vi "rszvl_core_global.vi"() -> ()   [LabVIEW 2014] (continued)
"*WAI"=FALSE}, "Check Status Callback"=""}, {"Level"=2, "Descriptive Name"="Time Trigger", "Class Only"=TRUE, "Data Type"=0, "Access"=0, "Identifier"="", "Range Table"="", "Command"="", "Read Callback"="", "Write Callback"="", "Range Callback"="", "Check Callback"="", "Rngtable Callback"="", "Coerce Callback"="", "User Callback"="", "Supported Models"="", "Instrument Options"="", "Repeated Capabilities"="", "Restricted Repeated Capabilities"="", "Help"="Time Trigger configuration.\n\n(1) Time Interval:\nThis attribute sets the time intervall for the time trigger source.", "Flags"={"OPC Wait"=FALSE, "Dont check status"=FALSE, "*WAI"=FALSE}, "Check Status Callback"=""}, {"Level"=3, "Descriptive Name"="Time Interval", "Class Only"=FALSE, "Data Type"=1, "Access"=2, "Identifier"="RSZVL_ATTR_TRIGGER_TIME_INTERVAL", "Range Table"="rszvl_rngTriggerTimeInterval", "Command"="TRIG:TIME:RINT", "Read Callback"="", "Write Callback"="", "Range Callback"="", "Check Callback"="", "Rngtable Callback"="", "Coerce Callback"="", "User Callback"="", "Supported Models"="", "Instrument Options"="", "Repeated Capabilities"="", "Restricted Repeated Capabilities"="", "Help"="This attribute sets the time intervall for the time trigger source.\n\nAvailable Repeated Capabilities:\nNone\n\nRemote-control command(s):\nTRIGger<1|2>[:SEQuence]:TIME:RINTerval", "Flags"={"OPC Wait"=FALSE, "Dont check status"=FALSE, "*WAI"=FALSE}, "Check Status Callback"=""}, {"Level"=1, "Descriptive Name"="Amplitude", "Class Only"=TRUE, "Data Type"=0, "Access"=0, "Identifier"="", "Range Table"="", "Command"="", "Read Callback"="", "Write Callback"="", "Range Callback"="", "Check Callback"="", "Rngtable Callback"="", "Coerce Callback"="", "User Callback"="", "Supported Models"="", "Instrument Options"="", "Repeated Capabilities"="", "Restricted Repeated Capabilities"="", "Help"="(1) Amplitude Preamplifier State:\nThis attribute switches on the preamplifier for the instrument. The switchable gain is fixed to 20 dB.", "Flags"={"OPC Wait"=FALSE, "Dont check status"=FALSE, "*WAI"=FALSE}, "Check Status Callback"=""}, {"Level"=2, "Descriptive Name"="Amplitude Preamplifier State", "Class Only"=FALSE, "Data Type"=3, "Access"=2, "Identifier"="RSZVL_ATTR_AMPL_PREAMPLIFIER", "Range Table"="", "Command"="INP:GAIN:STAT", "Read Callback"="", "Write Callback"="", "Range Callback"="", "Check Callback"="", "Rngtable Callback"="", "Coerce Callback"="", "User Callback"="", "Supported Models"="", "Instrument Options"="", "Repeated Capabilities"="", "Restricted Repeated Capabilities"="", "Help"="This attribute switches on the preamplifier for the instrument. The switchable gain is fixed to 20 dB.\n\nAvailable Repeated Capabilities:\nNone\n\nRemote-control command(s):\nINPut<1|2>:GAIN:STATe ON | OFF", "Flags"={"OPC Wait"=FALSE, "Dont check status"=FALSE, "*WAI"=FALSE}, "Check Status Callback"=""}, {"Level"=1, "Descriptive Name"="Measurement", "Class Only"=TRUE, "Data Type"=0, "Access"=0, "Identifier"="", "Range Table"="", "Command"="", "Read Callback"="", "Write Callback"="", "Range Callback"="", "Check Callback"="", "Rngtable Callback"="", "Coerce Callback"="", "User Callback"="", "Supported Models"="", "Instrument Options"="", "Repeated Capabilities"="", "Restricted Repeated Capabilities"="", "Help"="(1) Limit Check Result:\nThis attribute queries the result of the limit check of the limit line indicated. It should be noted that a complete sweep must have been performed for obtaining a valid result. A synchronization with  *OPC, *OPC? or *WAI should therefore be provided.\nThe result of the limit check responds with 0 for PASS, 1 for FAIL, and 2 for MARGIN.\n\n(2) Noise (Class):\nNoise measurement configuration and results.\n\n(3) Phase Noise (Class):\nPhase Noise measurement configuration and results.\n\n(4) Signal Count (Class):\nSignal count measurement configuration and results.\n\n(5) n dB Down (Class):\nn dB Down marker measurement configuration and results.\n\n(6) List Power (Class):\nList Power measurement configuration and results.\n\n(7) Time Domain Power (Class):\nTime Domain Power measurement configuration and results.\n\n(8) Power Measurements (Class):\nPower measurement configuration and results.\n\n(9) Signal Statistic (Class):\nSignal Statistic measurement configuration and results.\n\n(10) Modulation Depth (Class):\nModulation Depth measurement configuration and results.\n\n(11) Third Order Intercept (Class):\nThird Order Intercept measurement configuration and results.\n\n(12) Harmonic Distortion (Class):\nHarmonic Distortion measurement configuration and results.\n\n(13) Burst Power (Class):\nBurst Power measurement configuration and results.\n\n(14) IQ Measurement (Class):\nIQ  measurement configuration and results.", "Flags"={"OPC Wait"=FALSE, "Dont check status"=FALSE, "*WAI"=FALSE}, "Check Status Callback"=""}, {"Level"=2, "Descriptive Name"="Limit Check Result", "Class Only"=FALSE, "Data Type"=0, "Access"=0, "Identifier"="RSZVL_LIMIT_CHECK_RESULT", "Range Table"="", "Command"="CALC:LIM{Limit}:FAIL?", "Read Callback"="", "Write Callback"="", "Range Callback"="", "Check Callback"="", "Rngtable Callback"="", "Coerce Callback"="", "User Callback"="", "Supported Models"="", "Instrument Options"="", "Repeated Capabilities"="", "Restricted Repeated Capabilities"="", "Help"="This attribute queries the result of the limit check of the limit line indicated. It should be noted that a complete sweep must have been performed for obtaining a valid result. A synchronization with  *OPC, *OPC? or *WAI should therefore be provided.\nThe result of the limit check responds with 0 for PASS, 1 for FAIL, and 2 for MARGIN.\n\nAvailable Repeated Capabilities:\nLimit: L1,L2,L3,L4,L5,L6,L7,L8\r\n\nRemote-control command(s):\nCALCulate<1|2>:LIMit<1 to 8>:FAIL?", "Flags"={"OPC Wait"=FALSE, "Dont check status"=FALSE, "*WAI"=FALSE}, "Check Status Callback"=""}, {"Level"=2, "Descriptive Name"="Noise", "Class Only"=TRUE, "Data Type"=0, "Access"=0, "Identifier"="", "Range Table"="", "Command"="", "Read Callback"="", "Write Callback"="", "Range Callback"="", "Check Callback"="", "Rngtable Callback"="", "Coerce Callback"="", "User Callback"="", "Supported Models"="", "Instrument Options"="", "Repeated Capabilities"="", "Restricted Repeated Capabilities"="", "Help"="Noise measurement configuration and results.", "Flags"={"OPC Wait"=FALSE, "Dont check status"=FALSE, "*WAI"=FALSE}, "Check Status Callback"=""}, {"Level"=3, "Descriptive Name"="Marker Noise Measurement State", "Class Only"=FALSE, "Data Type"=3, "Access"=2, "Identifier"="RSZVL_ATTR_MARKER_NOISE_STATE", "Range Table"="", "Command"="CALC:MARK{Marker}:FUNC:NOIS", "Read Callback"="", "Write Callback"="", "Range Callback"="", "Check Callback"="", "Rngtable Callback"="", "Coerce Callback"="", "User Callback"="", "Supported Models"="", "Instrument Options"="", "Repeated Capabilities"="", "Restricted Repeated Capabilities"="", "Help"="This attribute switches the noise measurement on or off for all markers. The noise power density is measured at the position of the markers.\n\nAvailable Repeated Capabilities:\nMarker: M1,M2,M3,M4\r\n\nRemote-control command(s):\nCALCulate<1|2>:MARKer<1 to 4>:FUNCtion:NOISe[:STATe] ON | OFF", "Flags"={"OPC Wait"=FALSE, "Dont check status"=FALSE, "*WAI"=FALSE}, "Check Status Callback"=""}, {"Level"=3, "Descriptive Name"="Marker Noise Measurement Result", "Class Only"=FALSE, "Data Type"=1, "Access"=0, "Identifier"="RSZVL_ATTR_MARKER_NOISE_RESULT", "Range Table"="", "Command"="CALC:MARK{Marker}:FUNC:NOIS:RES?", "Read Callback"="", "Write Callback"="", "Range Callback"="", "Check Callback"="", "Rngtable Callback"="", "Coerce Callback"="", "User Callback"="", "Supported Models"="", "Instrument Options"="", "Repeated Capabilities"="", "Restricted Repeated Capabilities"="", "Help"="This attribute queries the result of the noise measurement.\nA complete sweep with synchronization to the sweep end must be performed between switching on the function and querying the measured value in order to obtain a valid query result. This is only possible in single sweep mode.\n\nAvailable Repeated Capabilities:\nMarker: M1,M2,M3,M4\r\n\nRemote-control command(s):\nCALCulate<1|2>:MARKer<1 to 4>:FUNCtion:NOISe:RESult?", "Flags"={"OPC Wait"=FALSE, "Dont check status"=FALSE, "*WAI"=FALSE}, "Check Status Callback"=""}, {"Level"=2, "Descriptive Name"="Phase Noise", "Class Only"=TRUE, "Data Type"=0, "Access"=0, "Identifier"="", "Range Table"="", "Command"="", "Read Callback"="", "Write Callback"="", "Range Callback"="", "Check Callback"="", "Rngtable Callback"="", "Coerce Callback"="", "User Callback"="", "Supported Models"="", "Instrument Options"="", "Repeated Capabilities"="", "Restricted Repeated Capabilities"="", "Help"="Phase Noise measurement configuration and results.", "Flags"={"OPC Wait"=FALSE, "Dont check status"=FALSE, "*WAI"=FALSE}, "Check Status Callback"=""}, {"Level"=3, "Descriptive Name"="Delta Marker Phase Noise State", "Class Only"=FALSE, "Data Type"=3, "Access"=2, "Identifier"="RSZVL_ATTR_REFERENCE_MARKER_PNO_STATE", "Range Table"="", "Command"="CALC:DELT:FUNC:PNO", "Read Callback"="", "Write Callback"="", "Range Callback"="", "Check Callback"="", "Rngtable Callback"="", "Coerce Callback"="", "User Callback"="", "Supported Models"="", "Instrument Options"="", "Repeated Capabilities"="", "Restricted Repeated Capabilities"="", "Help"="This attribute switches on or off the phase-noise measurement with all active delta markers. The correction values for the bandwidth and the log amplifier are taken into account in the measurement.\nMarker 1 will be activated, if necessary, and a peak search will be performed. If marker 1 is activated, its position becomes the reference point for the measurement.\nThe reference point can then be modified with commands CALCulate:DELTamarker:FUNCtion:FIXed:RPOint:X and ...:RPOint:Y independently of the position of marker 1 and of a trace (the same commands used for the measurment with fixed reference point).\n\nAvailable Repeated Capabilities:\nNone\n\nRemote-control command(s):\nCALCulate<1|2>:DELTamarker<1 to 4>:FUNCtion:PNOise[:STATe] ON | OFF", "Flags"={"OPC Wait"=FALSE, "Dont check status"=FALSE, "*WAI"=FALSE}, "Check Status Callback"=""}, {"Level"=3, "Descriptive Name"="Delta Marker Phase Noise Result", "Class Only"=FALSE, "Data Type"=1, "Access"=0, "Identifier"="RSZVL_ATTR_REFERENCE_MARKER_PNO_RESULT", "Range Table"="", "Command"="CALC:DELT:FUNC:PNO:RES?", "Read Callback"="", "Write Callback"="", "Range Callback"="", "Check Callback"="", "Rngtable Callback"="", "Coerce Callback"="", "User Callback"="", "Supported Models"="", "Instrument Options"="", "Repeated Capabilities"="", "Restricted Repeated Capabilities"="", "Help"="This attribute queries the result of the phase-noise measurement. The measurement will be switched on, if necessary.\n\nAvailable Repeated Capabilities:\nNone\n\nRemote-control command(s):\nCALCulate<1|2>:DELTamarker<1 to 4>:FUNCtion:PNOise:RESult?", "Flags"={"OPC Wait"=FALSE, "Dont check status"=FALSE, "*WAI"=FALSE}, "Check Status Callback"=""}, {"Level"=2, "Descriptive Name"="Signal Count", "Class Only"=TRUE, "Data Type"=0, "Access"=0, "Identifier"="", "Range Table"="", "Command"="", "Read Callback"="", "Write Callback"="", "Range Callback"="", "Check Callback"="", "Rngtable Callback"="", "Coerce Callback"="", "User Callback"="", "Supported Models"="", "Instrument Options"="", "Repeated Capabilities"="", "Restricted Repeated Capabilities"="", "Help"="Signal count measurement configuration and results.", "Flags"={"OPC Wait"=FALSE, "Dont check status"=FALSE, "*WAI"=FALSE}, "Check Status Callback"=""}, {"Level"=3, "Descriptive Name"="Frequency Counter State", "Class Only"=FALSE, "Data Type"=3, "Access"=2, "Identifier"="RSZVL_ATTR_MARKER_FREQUENCY_COUNTER_ENABLED", "Range Table"="", "Command"="CALC:MARK{Marker}:COUN", "Read Callback"="", "Write Callback"="", "Range Callback"="", "Check Callback"="", "Rngtable Callback"="", "Coerce Callback"="", "User Callback"="", "Supported Models"="", "Instrument Options"="", "Repeated Capabilities"="", "Restricted Repeated Capabilities"="", "Help"="This attribute switches on or off the frequency counter at the marker position.\nFrequency counting is possible only for one marker at a time. If it is activated for another marker, it is automatically de-activated for the previous marker. It should be noted that a complete sweep must be performed after switching on the frequency counter to ensure that the frequency to be measured is actually reached. The synchronization to the sweep end required for this is possible only in single-sweep mode.\n\nAvailable Repeated Capabilities:\nMarker: M1,M2,M3,M4\r\n\nRemote-control command(s):\nCALCulate<1|2>:MARKer<1 to 4>:COUNt ON | OFF", "Flags"={"OPC Wait"=FALSE, "Dont check status"=FALSE, "*WAI"=FALSE}, "Check Status Callback"=""}, {"Level"=3, "Descriptive Name"="Frequency Counter Resolution", "Class Only"=FALSE, "Data Type"=1, "Access"=2, "Identifier"="RSZVL_ATTR_MARKER_FREQUENCY_COUNTER_RESOLUTION", "Range Table"="rszvl_rngFreqCountRes", "Command"="CALC:MARK:COUN:RES", "Read Callback"="", "Write Callback"="", "Range Callback"="", "Check Callback"="", "Rngtable Callback"="", "Coerce Callback"="", "User Callback"="", "Supported Models"="", "Instrument Options"="", "Repeated Capabilities"="", "Restricted Repeated Capabilities"="", "Help"="This attribute specifies the resolution of the frequency counter. The setting is independent of the selected marker.\n\nAvailable Repeated Capabilities:\nNone\n\nRemote-control command(s):\nCALCulate<1|2>:MARKer<1 to 4>:COUNt:RESolution 0.1 | 1 | 10 | 100 | 1000 | 10000 Hz", "Flags"={"OPC Wait"=FALSE, "Dont check status"=FALSE, "*WAI"=FALSE}, "Check Status Callback"=""}, {"Level"=3, "Descriptive Name"="Frequency Counter Result", "Class Only"=FALSE, "Data Type"=1, "Access"=0, "Identifier"="RSZVL_ATTR_MARKER_COUNT", "Range Table"="", "Command"="CALC:MARK{Marker}:COUN:FREQ?", "Read Callback"="", "Write Callback"="", "Range Callback"="", "Check Callback"="", "Rngtable Callback"="", "Coerce Callback"="", "User Callback"="", "Supported Models"="", "Instrument Options"="", "Repeated Capabilities"="", "Restricted Repeated Capabilities"="", "Help"="This attribute queries the result of the frequency counter for the indicated marker. Before the command, the frequency counter should be switched on and a complete measurement performed to obtain a valid count result. Therefore, a single sweep with synchronization must be performed between switching on the frequency counter and querying the count result.\n\nAvailable Repeated Capabilities:\nMarker: M1,M2,M3,M4\r\n\nRemote-control command(s):\nCALCulate<1|2>:MARKer<1 to 4>:COUNt:FREQuency?", "Flags"={"OPC Wait"=FALSE, "Dont check status"=FALSE, "*WAI"=FALSE}, "Check Status Callback"=""}, {"Level"=2, "Descriptive Name"="n dB Down", "Class Only"=TRUE, "Data Type"=0, "Access"=0, "Identifier"="", "Range Table"="", "Command"="", "Read Callback"="", "Write Callback"="", "Range Callback"="", "Check Callback"="", "Rngtable Callback"="", "Coerce Callback"="", "User Callback"="", "Supported Models"="", "Instrument Options"="", "Repeated Capabilities"="", "Restricted Repeated Capabilities"="", "Help"="n dB Down marker measurement configuration and results.", "Flags"={"OPC Wait"=FALSE, "Dont check status"=FALSE, "*WAI"=FALSE}, "Check Status Callback"=""}, {"Level"=3, "Descriptive Name"="Marker N dB Down State", "Class Only"=FALSE, "Data Type"=3, "Access"=2, "Identifier"="RSZVL_ATTR_MARKER_NDB_STATE", "Range Table"="", "Command"="CALC:MARK:FUNC:NDBD:STAT", "Read Callback"="", "Write Callback"="", "Range Callback"="", "Check Callback"="", "Rngtable Callback"="", "Coerce Callback"="", "User Callback"="", "Supported Models"="", "Instrument Options"="", "Repeated Capabilities"="", "Restricted Repeated Capabilities"="", "Help"="This attribute switches the N dB Down function on or off. Marker 1 is activated first, if necessary.\n\nAvailable Repeated Capabilities:\nNone\n\nRemote-control command(s):\nCALCulate<1|2>:MARKer<1 to 4>:FUNCtion:NDBDown:STATe ON | OFF", "Flags"={"OPC Wait"=FALSE, "Dont check status"=FALSE, "*WAI"=FALSE}, "Check Status Callback"=""}, {"Level"=3, "Descriptive Name"="Marker N dB Down Value", "Class Only"=FALSE, "Data Type"=1, "Access"=2, "Identifier"="RSZVL_ATTR_MARKER_NDB_VAL", "Range Table"="rszvl_rngMarkerNdBDown", "Command"="CALC:MARK:FUNC:NDBD", "Read Callback"="", "Write Callback"="", "Range Callback"="", "Check Callback"="", "Rngtable Callback"="", "Coerce Callback"="", "User Callback"="", "Supported Models"="", "Instrument Options"="", "Repeated Capabilities"="", "Restricted Repeated Capabilities"="", "Help"="This attribute defines the level spacing of the two delta markers to the right and left of marker 1. Marker 1 is always used as the reference marker.\nThe temporary markers T1 and T2 are positioned by n dB below the active reference marker.\n\nAvailable Repeated Capabilities:\nNone\n\nRemote-control command(s):\nCALCulate<1|2>:MARKer<1 to 4>:FUNCtion:NDBDown", "Flags"={"OPC Wait"=FALSE, "Dont check status"=FALSE, "*WAI"=FALSE}, "Check Status Callback"=""}, {"Level"=3, "Descriptive Name"="Marker N dB Down Result", "Class Only"=FALSE, "Data Type"=1, "Access"=0, "Identifier"="RSZVL_ATTR_MARKER_NDB_RESULT", "Range Table"="", "Command"="CALC:MARK:FUNC:NDBD:RES?", "Read Callback"="", "Write Callback"="", "Range Callback"="", "Check Callback"="", "Rngtable Callback"="", "Coerce Callback"="", "User Callback"="", "Supported Models"="", "Instrument Options"="", "Repeated Capabilities"="", "Restricted Repeated Capabilities"="", "Help"="This attribute queries the frequency spacing (bandwidth) of the N-dB-down markers. A complete sweep with synchronization to sweep end must be performed between switching on the function and querying the measured value in order to obtain a valid query result. This is only possible in single sweep mode.\n\nAvailable Repeated Capabilities:\nNone\n\nRemote-control command(s):\nCALCulate<1|2>:MARKer<1 to 4>:FUNCtion:NDBDown:RESult?", "Flags"={"OPC Wait"=FALSE, "Dont check status"=FALSE, "*WAI"=FALSE}, "Check Status Callback"=""}, {"Level"=2, "Descriptive Name"="List Power", "Class Only"=TRUE, "Data Type"=0, "Access"=0, "Identifier"="", "Range Table"="", "Command"="", "Read Callback"="", "Write Callback"="", "Range Callback"="", "Check Callback"="", "Rngtable Callback"="", "Coerce Callback"="", "User Callback"="", "Supported Models"="", "Instrument Options"="", "Repeated Capabilities"="", "Restricted Repeated Capabilities"="", "Help"="List Power measurement configuration and results.", "Flags"={"OPC Wait"=FALSE, "Dont check status"=FALSE, "*WAI"=FALSE}, "Check Status Callback"=""}, {"Level"=3, "Descriptive Name"="List Power Measurement Deactivation", "Class Only"=FALSE, "Data Type"=4, "Access"=1, "Identifier"="RSZVL_ATTR_LIST_POW_STATE_OFF", "Range Table"="", "Command"="SENS:LIST:POW:STAT OFF", "Read Callback"="", "Write Callback"="", "Range Callback"="", "Check Callback"="", "Rngtable Callback"="", "Coerce Callback"="", "User Callback"="", "Supported Models"="", "Instrument Options"="", "Repeated Capabilities"="", "Restricted Repeated Capabilities"="", "Help"="This attribute deactivates the list measurement.\n\nAvailable Repeated Capabilities:\nNone\n\nRemote-control command(s):\n[SENSe<1|2>:]LIST:POWer:STATe OFF", "Flags"={"OPC Wait"=FALSE, "Dont check status"=FALSE, "*WAI"=FALSE}, "Check Status Callback"=""}, {"Level"=2, "Descriptive Name"="Time Domain Power", "Class Only"=TRUE, "Data Type"=0, "Access"=0, "Identifier"="", "Range Table"="", "Command"="", "Read Callback"="", "Write Callback"="", "Range Callback"="", "Check Callback"="", "Rngtable Callback"="", "Coerce Callback"="", "User Callback"="", "Supported Models"="", "Instrument Options"="", "Repeated Capabilities"="", "Restricted Repeated Capabilities"="", "Help"="Time Domain Power measurement configuration and results.", "Flags"={"OPC Wait"=FALSE, "Dont check status"=FALSE, "*WAI"=FALSE}, "Check Status Callback"=""}, {"Level"=3, "Descriptive Name"="Time Domain Power State", "Class Only"=FALSE, "Data Type"=3, "Access"=2, "Identifier"="RSZVL_ATTR_MEAS_TDOM_STATE", "Range Table"="", "Command"="CALC:MARK:FUNC:SUMM", "Read Callback"="", "Write Callback"="", "Range Callback"="", "Check Callback"="", "Rngtable Callback"="", "Coerce Callback"="", "User Callback"="", "Supported Models"="", "Instrument Options"="", "Repeated Capabilities"="", "Restricted Repeated Capabilities"="", "Help"="This attribute switches on or off the previously selected time domain power measurements. Thus one or several measurements can be first selected and then switched on and off together with this attribute.\nThe function is independent of the marker selection. It is only available in the time domain (span = 0).\n\nAvailable Repeated Capabilities:\nNone\n\nRemote-control command(s):\nCALCulate<1|2>:MARKer<1 to 4>:FUNCtion:SUMMary[:STATe] ON | OFF", "Flags"={"OPC Wait"=FALSE, "Dont check status"=FALSE, "*WAI"=FALSE}, "Check Status Callback"=""}, {"Level"=3, "Descriptive Name"="Time Domain Power Peak State", "Class Only"=FALSE, "Data Type"=3, "Access"=2, "Identifier"="RSZVL_ATTR_MEAS_TDOM_PEAK", "Range Table"="", "Command"="CALC:MARK:FUNC:SUMM:PPE", "Read Callback"="", "Write Callback"="", "Range Callback"="", "Check Callback"="", "Rngtable Callback"="", "Coerce Callback"="", "User Callback"="", "Supported Models"="", "Instrument Options"="", "Repeated Capabilities"="", "Restricted Repeated Capabilities"="", "Help"="This attribute switches on or off the measurement of the positive peak value.\nThe function is independent of the marker selection. It is only available in the time domain (span = 0).\n\nAvailable Repeated Capabilities:\nNone\n\nRemote-control command(s):\nCALCulate<1|2>:MARKer<1 to 4>:FUNCtion:SUMMary:PPEak[:STATe] ON | OFF", "Flags"={"OPC Wait"=FALSE, "Dont check status"=FALSE, "*WAI"=FALSE}, "Check Status Callback"=""}, {"Level"=3, "Descriptive Name"="Time Domain Power RMS State", "Class Only"=FALSE, "Data Type"=3, "Access"=2, "Identifier"="RSZVL_ATTR_MEAS_TDOM_RMS", "Range Table"="", "Command"="CALC:MARK:FUNC:SUMM:RMS", "Read Callback"="", "Write Callback"="", "Range Callback"="", "Check Callback"="", "Rngtable Callback"="", "Coerce Callback"="", "User Callback"="", "Supported Models"="", "Instrument Options"="", "Repeated Capabilities"="", "Restricted Repeated Capabilities"="", "Help"="This attribute switches on or off the measurement of the effective (RMS) power. If necessary the function is switched on previously.\nThe function is independent of the marker selection. It is only available in the time domain (span = 0).\n\nAvailable Repeated Capabilities:\nNone\n\nRemote-control command(s):\nCALCulate<1|2>:MARKer<1 to 4>:FUNCtion:SUMMary:RMS[:STATe] ON | OFF", "Flags"={"OPC Wait"=FALSE, "Dont check status"=FALSE, "*WAI"=FALSE}, "Check Status Callback"=""}, {"Level"=3, "Descriptive Name"="Time Domain Power Mean State", "Class Only"=FALSE, "Data Type"=3, "Access"=2, "Identifier"="RSZVL_ATTR_MEAS_TDOM_MEAN", "Range Table"="", "Command"="CALC:MARK:FUNC:SUMM:MEAN", "Read Callback"="", "Write Callback"="", "Range Callback"="", "Check Callback"="", "Rngtable Callback"="", "Coerce Callback"="", "User Callback"="", "Supported Models"="", "Instrument Options"="", "Repeated Capabilities"="", "Restricted Repeated Capabilities"="", "Help"="This attribute switches on or off the measurement of the mean value.\nThe function is independent of the marker selection. It is only available in the time domain (span = 0).\n\nNote(s):\n(1) The measurement is performed on the trace on which marker 1 is positioned. In order to evaluate another trace, marker 1 must be positioned on another trace.\n\nAvailable Repeated Capabilities:\nNone\n\nRemote-control command(s):\nCALCulate<1|2>:MARKer<1 to 4>:FUNCtion:SUMMary:MEAN[:STATe] ON | OFF", "Flags"={"OPC Wait"=FALSE, "Dont check status"=FALSE, "*WAI"=FALSE}, "Check Status Callback"=""}, {"Level"=3, "Descriptive Name"="Time Domain Power Standard Deviation State", "Class Only"=FALSE, "Data Type"=3, "Access"=2, "Identifier"="RSZVL_ATTR_MEAS_TDOM_SDEV", "Range Table"="", "Command"="CALC:MARK:FUNC:SUMM:SDEV", "Read Callback"="", "Write Callback"="", "Range Callback"="", "Check Callback"="", "Rngtable Callback"="", "Coerce Callback"="", "User Callback"="", "Supported Models"="", "Instrument Options"="", "Repeated Capabilities"="", "Restricted Repeated Capabilities"="", "Help"="This command switches on or off the measurement of the standard deviation.\nThe function is independent of the marker selection. It is only available in the time domain (span = 0).\n\nNote(s):\n(1) On switching on the measurement, the mean power measurement is switched on as well.\n\nAvailable Repeated Capabilities:\nNone\n\nRemote-control command(s):\nCALCulate<1|2>:MARKer<1 to 4>:FUNCtion:SUMMary:SDEViation[:STATe] ON | OFF", "Flags"={"OPC Wait"=FALSE, "Dont check status"=FALSE, "*WAI"=FALSE}, "Check Status Callback"=""}, {"Level"=3, "Descriptive Name"="Time Domain Power Average", "Class Only"=FALSE, "Data Type"=3, "Access"=2, "Identifier"="RSZVL_ATTR_MEAS_TDOM_AVG", "Range Table"="", "Command"="CALC:MARK:FUNC:SUMM:AVER", "Read Callback"="", "Write Callback"="", "Range Callback"="", "Check Callback"="", "Rngtable Callback"="", "Coerce Callback"="", "User Callback"="", "Supported Models"="", "Instrument Options"="", "Repeated Capabilities"="", "Restricted Repeated Capabilities"="", "Help"="This attribute switches on or off averaging for the active time domain power measurement. The function is independent of the marker selection. It is only available in the time domain (span = 0).\nAveraging is reset by switching it off and on again.\nIt should be noted that synchronization to the end of averaging is only possible in single sweep mode.\n\nAvailable Repeated Capabilities:\nNone\n\nRemote-control command(s):\nCALCulate<1|2>:MARKer<1 to 4>:FUNCtion:SUMMary:AVERage ON | OFF", "Flags"={"OPC Wait"=FALSE, "Dont check status"=FALSE, "*WAI"=FALSE}, "Check Status Callback"=""}, {"Level"=3, "Descriptive Name"="Time Domain Power Max Hold", "Class Only"=FALSE, "Data Type"=3, "Access"=2, "Identifier"="RSZVL_ATTR_MEAS_TDOM_MAX_HOLD", "Range Table"="", "Command"="CALC:MARK:FUNC:SUMM:PHOL", "Read Callback"="", "Write Callback"="", "Range Callback"="", "Check Callback"="", "Rngtable Callback"="", "Coerce Callback"="", "User Callback"="", "Supported Models"="", "Instrument Options"="", "Repeated Capabilities"="", "Restricted Repeated Capabilities"="", "Help"="This attribute switches on or off the peak-hold function for the active time domain power measurement. The function is independent of the marker selection. It is only available in the time domain (span = 0).\nThe peak-hold function is reset by switching it off and on again.\n\nAvailable Repeated Capabilities:\nNone\n\nRemote-control command(s):\nCALCulate<1|2>:MARKer<1 to 4>:FUNCtion:SUMMary:PHOLd ON | OFF", "Flags"={"OPC Wait"=FALSE, "Dont check status"=FALSE, "*WAI"=FALSE}, "Check Status Callback"=""}, {"Level"=3, "Descriptive Name"="Time Domain Power Mode", "Class Only"=FALSE, "Data Type"=0, "Access"=2, "Identifier"="RSZVL_ATTR_MEAS_TDOM_MODE", "Range Table"="rszvl_rngAbsRel", "Command"="CALC:MARK:FUNC:SUMM:MODE", "Read Callback"="", "Write Callback"="", "Range Callback"="", "Check Callback"="", "Rngtable Callback"="", "Coerce Callback"="", "User Callback"="", "Supported Models"="", "Instrument Options"="", "Repeated Capabilities"="", "Restricted Repeated Capabilities"="", "Help"="This attribute selects absolute or relative time domain power measurement. The function is independent of the marker selection. It is only available in the time domain (span = 0).\nIf the reference power is not defined, the value 0 dBm is used.\n\nAvailable Repeated Capabilities:\nNone\n\nRemote-control command(s):\nCALCulate<1|2>:MARKer<1 to 4>:FUNCtion:SUMMary:MODE ABSolute | RELative", "Flags"={"OPC Wait"=FALSE, "Dont check status"=FALSE, "*WAI"=FALSE}, "Check Status Callback"=""}, {"Level"=3, "Descriptive Name"="Time Domain Power All Off", "Class Only"=FALSE, "Data Type"=4, "Access"=1, "Identifier"="RSZVL_ATTR_MEAS_TDOM_AOFF", "Range Table"="", "Command"="CALC:MARK:FUNC:SUMM:AOFF", "Read Callback"="", "Write Callback"="", "Range Callback"="", "Check Callback"="", "Rngtable Callback"="", "Coerce Callback"="", "User Callback"="", "Supported Models"="", "Instrument Options"="", "Repeated Capabilities"="", "Restricted Repeated Capabilities"="", "Help"="This attribute switches off all time domain measurements. The function is independent of the marker selection. It is only available in the time domain (span = 0).\n\nAvailable Repeated Capabilities:\nNone\n\nRemote-control command(s):\nCALCulate<1|2>:MARKer<1 to 4>:FUNCtion:SUMMary:AOFF", "Flags"={"OPC Wait"=FALSE, "Dont check status"=FALSE, "*WAI"=FALSE}, "Check Status Callback"=""}, {"Level"=3, "Descriptive Name"="Time Domain Power Set Reference", "Class Only"=FALSE, "Data Type"=4, "Access"=1, "Identifier"="RSZVL_ATTR_MEAS_TDOM_SET_REFERENCE", "Range Table"="", "Command"="*WAI;:CALC:MARK:FUNC:SUMM:REF:AUTO ONCE", "Read Callback"="", "Write Callback"="", "Range Callback"="", "Check Callback"="", "Rngtable Callback"="", "Coerce Callback"="", "User Callback"="", "Supported Models"="", "Instrument Options"="", "Repeated Capabilities"="", "Restricted Repeated Capabilities"="", "Help"="With this attribute the currently measured average value and RMS value are declared as reference values for relative measurements. The function is independent of the marker selection. It is only available in the time domain (span = 0).\nIf the function of Averaging or Peak Hold is switched on, the current value is the accumulated measurement value at the time considered.\n\nNote(s):\n\n(1) This attribute sends *WAI command\n\nAvailable Repeated Capabilities:\nNone\n\nRemote-control command(s):\nCALCulate<1|2>:MARKer<1 to 4>:FUNCtion:SUMMary:REFerence:AUTO ONCE", "Flags"={"OPC Wait"=FALSE, "Dont check status"=FALSE, "*WAI"=FALSE}, "Check Status Callback"=""}, {"Level"=3, "Descriptive Name"="Time Domain Power Peak Result", "Class Only"=FALSE, "Data Type"=1, "Access"=0, "Identifier"="RSZVL_ATTR_MEAS_TDOM_PEAK_RESULT", "Range Table"="", "Command"="CALC:MARK:FUNC:SUMM:PPE:RES?", "Read Callback"="", "Write Callback"="", "Range Callback"="", "Check Callback"="", "Rngtable Callback"="", "Coerce Callback"="", "User Callback"="", "Supported Models"="", "Instrument Options"="", "Repeated Capabilities"="", "Restricted Repeated Capabilities"="", "Help"="This attribute is used to query the result of the measurement of the positive peak value. The measurement may have to be switched on previously.\nThe function is independent of the marker selection. It is only available in the time domain (span = 0).\nA complete sweep with synchronization to sweep end must be performed between switching on the function and querying the measured value to obtain a valid query result. This is only possible in single sweep mode.\n\nAvailable Repeated Capabilities:\nNone\n\nRemote-control command(s):\nCALCulate<1|2>:MARKer<1 to 4>:FUNCtion:SUMMary:PPEak:RESult?", "Flags"={"OPC Wait"=FALSE, "Dont check status"=FALSE, "*WAI"=FALSE}, "Check Status Callback"=""}, {"Level"=3, "Descriptive Name"="Time Domain Power RMS Result", "Class Only"=FALSE, "Data Type"=1, "Access"=0, "Identifier"="RSZVL_ATTR_MEAS_TDOM_RMS_RESULT", "Range Table"="", "Command"="CALC:MARK:FUNC:SUMM:RMS:RES?", "Read Callback"="", "Write Callback"="", "Range Callback"="", "Check Callback"="", "Rngtable Callback"="", "Coerce Callback"="", "User Callback"="", "Supported Models"="", "Instrument Options"="", "Repeated Capabilities"="", "Restricted Repeated Capabilities"="", "Help"="This attribute queries the result of the measurement of the RMS power value.\nThe function is independent of the marker selection. It is only available in the time domain (span = 0).\nA complete sweep with synchronization to sweep end must be performed between switching on the function and querying the measured value to obtain a valid query result. This is only possible in single sweep mode.\n\nAvailable Repeated Capabilities:\nNone\n\nRemote-control command(s):\nCALCulate<1|2>:MARKer<1 to 4>:FUNCtion:SUMMary:RMS:RESult?", "Flags"={"OPC Wait"=FALSE, "Dont check status"=FALSE, "*WAI"=FALSE}, "Check Status Callback"=""}, {"Level"=3, "Descriptive Name"="Time Domain Power Mean Result", "Class Only"=FALSE, "Data Type"=1, "Access"=0, "Identifier"="RSZVL_ATTR_MEAS_TDOM_MEAN_RESULT", "Range Table"="", "Command"="CALC:MARK:FUNC:SUMM:MEAN:RES?", "Read Callback"="", "Write Callback"="", "Range Callback"="", "Check Callback"="", "Rngtable Callback"="", "Coerce Callback"="", "User Callback"="", "Supported Models"="", "Instrument Options"="", "Repeated Capabilities"="", "Restricted Repeated Capabilities"="", "Help"="This attribute queries the result of the measurement of the mean value.\nThe function is independent of the marker selection. It is only available in the time domain (span = 0).\nA complete sweep with synchronization to sweep end must be performed between switching on the function and querying the measured value to obtain a valid query result. This is only possible in single sweep mode.\n\nAvailable Repeated Capabilities:\nNone\n\nRemote-control command(s):\nCALCulate<1|2>:MARKer<1 to 4>:FUNCtion:SUMMary:MEAN:RESult?", "Flags"={"OPC Wait"=FALSE, "Dont check status"=FALSE, "*WAI"=FALSE}, "Check Status Callback"=""}, {"Level"=3, "Descriptive Name"="Time Domain Power Standard Deviation Result", "Class Only"=FALSE, "Data Type"=1, "Access"=0, "Identifier"="RSZVL_ATTR_MEAS_TDOM_SDEV_RESULT", "Range Table"="", "Command"="CALC:MARK:FUNC:SUMM:SDEV:RES?", "Read Callback"="", "Write Callback"="", "Range Callback"="", "Check Callback"="", "Rngtable Callback"="", "Coerce Callback"="", "User Callback"="", "Supported Models"="", "Instrument Options"="", "Repeated Capabilities"="", "Restricted Repeated Capabilities"="", "Help"="This attribute queries the results of the standard deviation measurement.\nThe function is independent of the marker selection. It is only available in the time domain (span = 0).\nA complete sweep with synchronization to sweep end must be performed between switching on the function and querying the measured value to obtain a valid query result. This is only possible in single sweep mode.\n\nAvailable Repeated Capabilities:\nNone\n\nRemote-control command(s):\nCALCulate<1|2>:MARKer<1 to 4>:FUNCtion:SUMMary:SDEViation:RESult?", "Flags"={"OPC Wait"=FALSE, "Dont check status"=FALSE, "*WAI"=FALSE}, "Check Status Callback"=""}, {"Level"=3, "Descriptive Name"="Time Domain Power Averaged Peak Result", "Class Only"=FALSE, "Data Type"=1, "Access"=0, "Identifier"="RSZVL_ATTR_MEAS_TDOM_AVG_PEAK_RESULT", "Range Table"="", "Command"="CALC:MARK:FUNC:SUMM:PPE:AVER:RES?", "Read Callback"="", "Write Callback"="", "Range Callback"="", "Check Callback"="", "Rngtable Callback"="", "Coerce Callback"="", "User Callback"="", "Supported Models"="", "Instrument Options"="", "Repeated Capabilities"="", "Restricted Repeated Capabilities"="", "Help"="This attribute is used to query the result of the measurement of the averaged positive peak value. The query is only possible if averaging has been activated previously.\nThe function is independent of the marker selection. It is only available in the time domain (span = 0).\nA complete sweep with synchronization to sweep end must be performed between switching on the function and querying the measured value to obtain a valid query result. This is only possible in single sweep mode.\n\nAvailable Repeated Capabilities:\nNone\n\nRemote-control command(s):\nCALCulate<1|2>:MARKer<1 to 4>:FUNCtion:SUMMary:PPEak:AVERage:RESult?", "Flags"={"OPC Wait"=FALSE, "Dont check status"=FALSE, "*WAI"=FALSE}, "Check Status Callback"=""}, {"Level"=3, "Descriptive Name"="Time Domain Power Averaged RMS Result", "Class Only"=FALSE, "Data Type"=1, "Access"=0, "Identifier"="RSZVL_ATTR_MEAS_TDOM_AVG_RMS_RESULT", "Range Table"="", "Command"="CALC:MARK:FUNC:SUMM:RMS:AVER:RES?", "Read Callback"="", "Write Callback"="", "Range Callback"="", "Check Callback"="", "Rngtable Callback"="", "Coerce Callback"="", "User Callback"="", "Supported Models"="", "Instrument Options"="", "Repeated Capabilities"="", "Restricted Repeated Capabilities"="", "Help"="This attribute queries the result of the measurement of the averaged RMS value. The query is only possible if averaging has been activated previously.\nThe function is independent of the marker selection. It is only available in the time domain (span = 0).\nA complete sweep with synchronization to sweep end must be performed between switching on the function and querying the measured value to obtain a valid query result. This is only possible in single sweep mode.\n\nAvailable Repeated Capabilities:\nNone\n\nRemote-control command(s):\nCALCulate<1|2>:MARKer<1 to 4>:FUNCtion:SUMMary:RMS:AVERage:RESult?", "Flags"={"OPC Wait"=FALSE, "Dont check status"=FALSE, "*WAI"=FALSE}, "Check Status Callback"=""}, {"Level"=3, "Descriptive Name"="Time Domain Power Averaged Mean Result", "Class Only"=FALSE, "Data Type"=1, "Access"=0, "Identifier"="RSZVL_ATTR_MEAS_TDOM_AVG_MEAN_RESULT", "Range Table"="", "Command"="CALC:MARK:FUNC:SUMM:MEAN:AVER:RES?", "Read Callback"="", "Write Callback"="", "Range Callback"="", "Check Callback"="", "Rngtable Callback"="", "Coerce Callback"="", "User Callback"="", "Supported Models"="", "Instrument Options"="", "Repeated Capabilities"="", "Restricted Repeated Capabilities"="", "Help"="This attribute queries the result of the measurement of the averaged mean value.\nThe query is only possible if averaging has been activated previously.\nThe function is independent of the marker selection. It is only available in the time domain (span = 0).\nA complete sweep with synchronization to sweep end must be performed between switching on the function and querying the measured value to obtain a valid query result. This is only possible in single sweep mode.\n\nAvailable Repeated Capabilities:\nNone\n\nRemote-control command(s):\nCALCulate<1|2>:MARKer<1 to 4>:FUNCtion:SUMMary:MEAN:AVERage:RESult?", "Flags"={"OPC Wait"=FALSE, "Dont check status"=FALSE, "*WAI"=FALSE}, "Check Status Callback"=""}, {"Level"=3, "Descriptive Name"="Time Domain Power Averaged Standard Deviation Result", "Class Only"=FALSE, "Data Type"=1, "Access"=0, "Identifier"="RSZVL_ATTR_MEAS_TDOM_AVG_SDEV_RESULT", "Range Table"="", "Command"="CALC:MARK:FUNC:SUMM:SDEV:AVER:RES?", "Read Callback"="", "Write Callback"="", "Range Callback"="", "Check Callback"="", "Rngtable Callback"="", "Coerce Callback"="", "User Callback"="", "Supported Models"="", "Instrument Options"="", "Repeated Capabilities"="", "Restricted Repeated Capabilities"="", "Help"="This attribute queries the result of the averaged standard deviation determined in several sweeps.\nThe query is only possible if averaging has been activated previously.\nThe function is independent of the marker selection. It is only available in the time domain (span = 0).\nA complete sweep with synchronization to sweep end must be performed between switching on the function and querying the measured value to obtain a valid query result. This is only possible in single sweep mode.\n\nAvailable Repeated Capabilities:\nNone\n\nRemote-control command(s):\nCALCulate<1|2>:MARKer<1 to 4>:FUNCtion:SUMMary:SDEViation:AVERage:RESult?", "Flags"={"OPC Wait"=FALSE, "Dont check status"=FALSE, "*WAI"=FALSE}, "Check Status Callback"=""}, {"Level"=3, "Descriptive Name"="Time Domain Power Peak Hold Result", "Class Only"=FALSE, "Data Type"=1, "Access"=0, "Identifier"="RSZVL_ATTR_MEAS_TDOM_PEAK_HOLD_RESULT", "Range Table"="", "Command"="CALC:MARK:FUNC:SUMM:PPE:PHOL:RES?", "Read Callback"="", "Write Callback"="", "Range Callback"="", "Check Callback"="", "Rngtable Callback"="", "Coerce Callback"="", "User 
